vi "setnag_testing.vi"() -> ()   [LabVIEW 2013]
doc: "This example demonstrates temperature control and monitoring.\n\nNote:\nBefore start this VI is it necessary:\n\n- preconfigure some specific parameters that are not supported by this driver (e.g. PV-I/O Type, Linearization type, Alarm Input Values... ) by Quick Codes, or by Eurotherm iTools or by instrument front panel controls\n- enter correct VISA Resource Descriptor, Device Address and Baud Rate into front-panel controls"
uses:
  <vilib>/DAQmx/read.llb/DAQmx Read (Analog DBL 1Chan 1Samp).vi
  <vilib>/Utility/file.llb/Write To Spreadsheet File (string).vi
  <vilib>/DAQmx/miscellaneous.llb/DAQmx Fill In Error Info.vi
panel:
  in  "stop":bool
  in  "Tab Control":enum32{"Setup", "QCM", "SetNag O2 Gauge"}(tab)
  in  "Add comments to the data file here and click anywhere outside the comment box to save. \nThe time at which comment is saved is recorded in the data file.":string
  out "Waveform Chart 2":dbl(graph)
  out "Waveform Chart":cluster{dbl}(graph)
  in  "Baud Rate":i32(ring)=2 items=["2400", "4800", "9600", "19200", "38400", "57600", "115200"]
  in  "Com Port":i32(ring) items=["Com 1", "Com 2", "Com 3", "Com 4", "Com 5", "Com 6", "COM 7", "COM 8", "COM 9", "COM 10", "COM 11", "COM 12", "com 13", "COM 14"]
  out "Torr":dbl
  out "%":dbl
  out "O2 pump voltage (V)":dbl format="%0.2f"
  out "atm":dbl
  # "Configuring Instrument\n \nPlease Wait......\n\nChart will update in 20 sec"
  # "Instructions:\n\nMake sure all instruments are plugged into the correct ports and all instruments are turned on.\n\nRun the Pirani Control software, and make sure the program is configured to save the temp / pressure / gas flow data. \n\nClick the RUN arrow on the toolbar, and wait for instruments to begin recording.\n\nTo end, click \"END PROGRAM AND SAVE DATA\". DO NOT press the STOP button on the toolbar."
  # "COMMENT BOX"
  # "BEFORE YOU RUN THIS VI:\n1. Turn on SetNag and get to 800C\n2. Turn on QCM and plug into corrent COM.\n3. Plug in USB DAQ 6008 and comment to SetNag"
  # "O2 Partial Pressure"
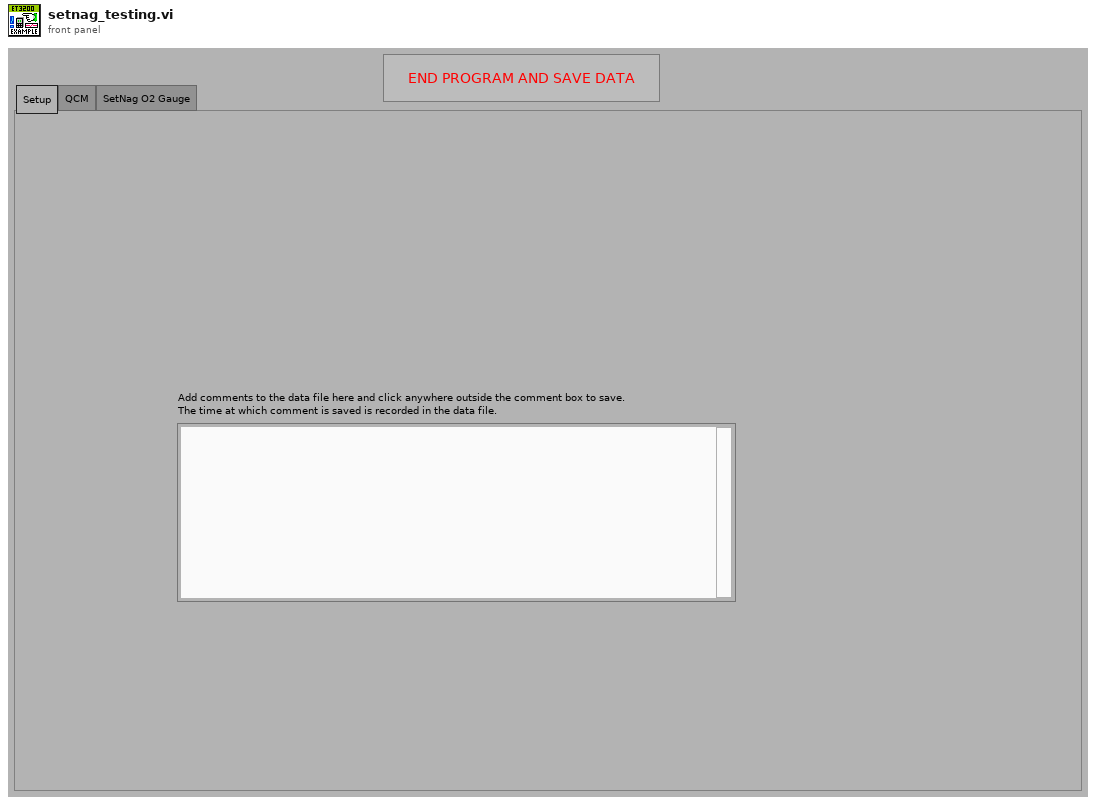
[diagram p1: front panel]
types:
  T1 = enum16{"no parity", "odd parity", "even parity", "mark parity", "space parity"}
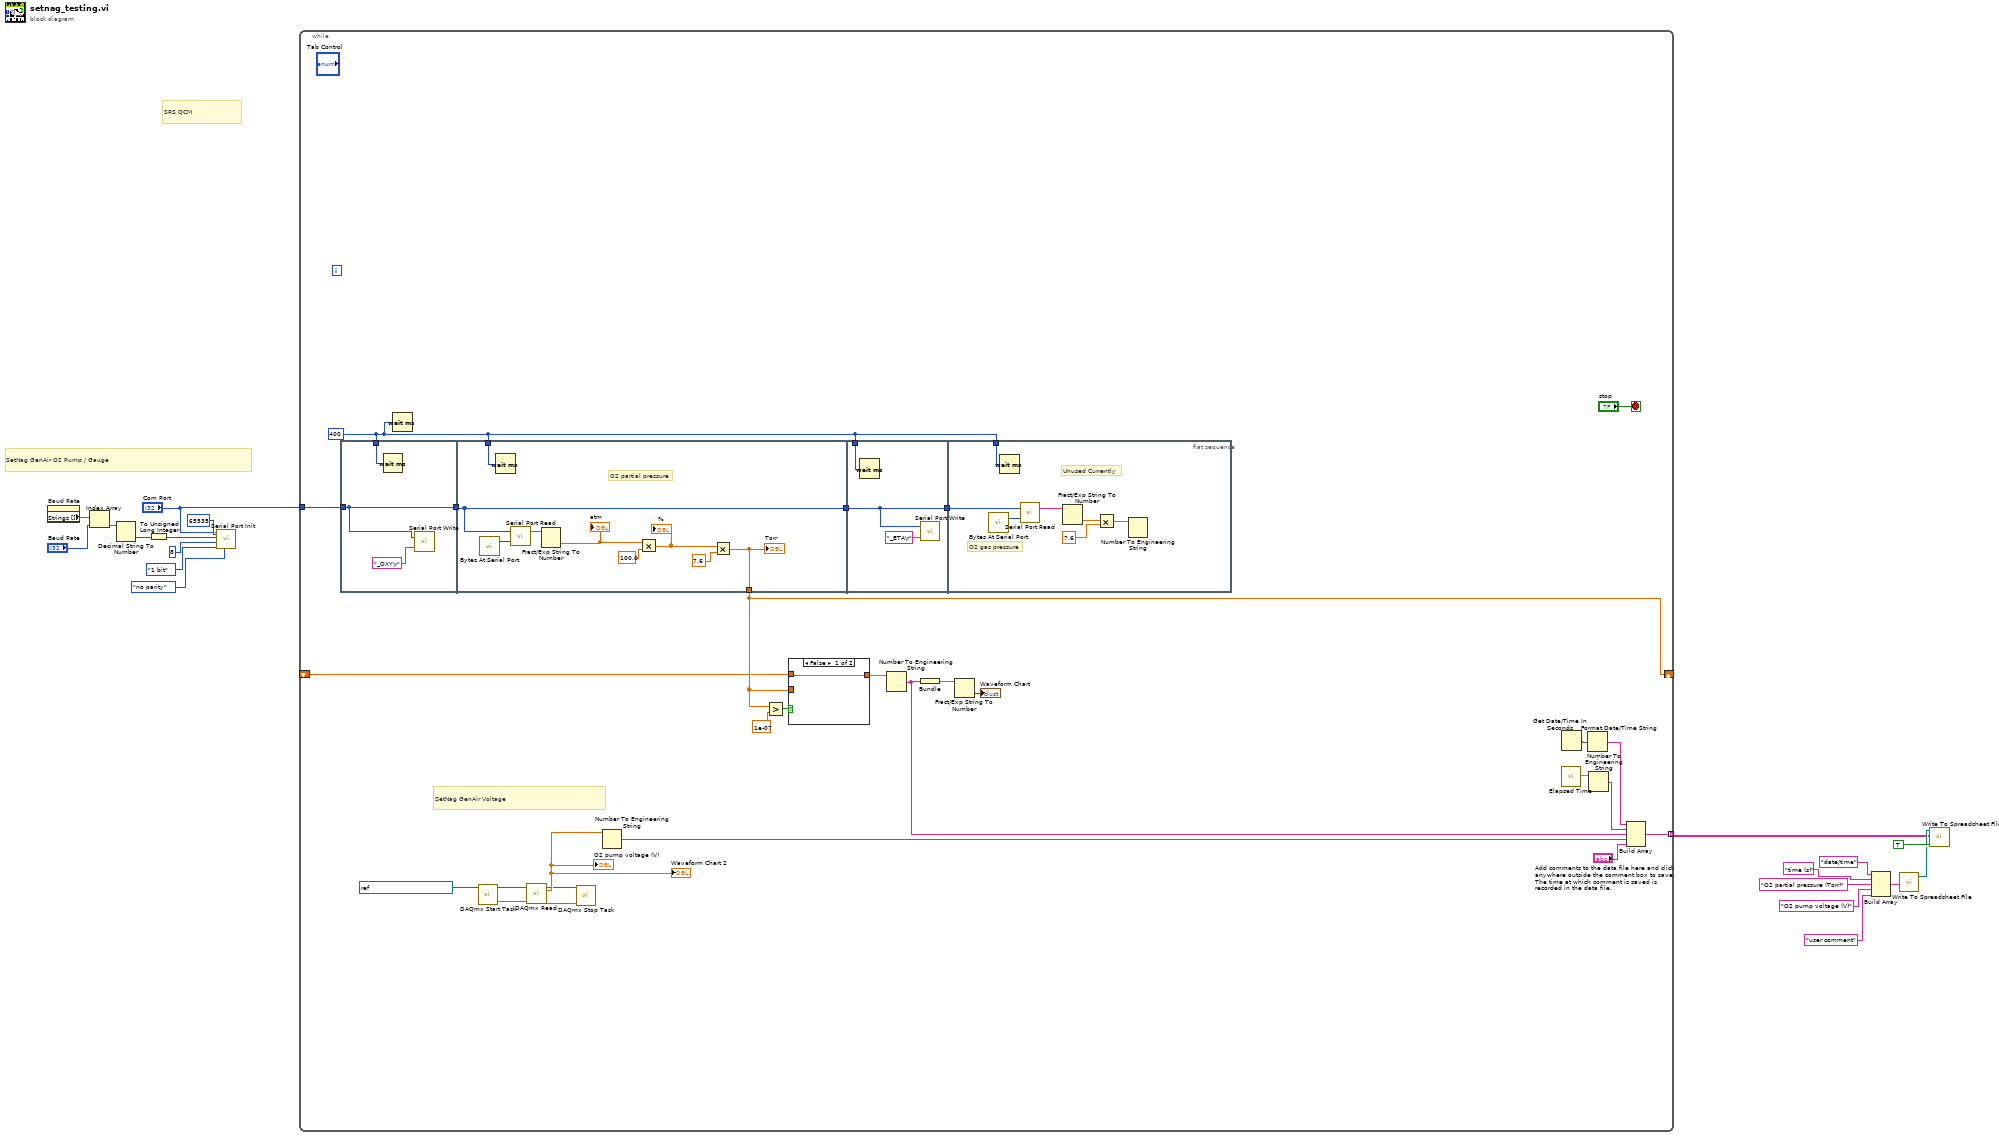
[diagram p0: block diagram]
diagram:
  # "SRS QCM"
  # "SetNag GenAir O2 Pump / Gauge"
  n1 = property on="Baud Rate" class="Ring (strict)"() -> ("Strings []"=w8:string[])  [unwired: 2 in, 2 out]
  n2 = Index Array(array=w8, index="Baud Rate") -> (element=w9:string)
  n3 = Decimal String To Number(string=w9) -> (number=w7:i32)  [unwired: 2 in, 1 out]
  n4 = To Unsigned Long Integer(number=w7) -> (unsigned 32bit integer=w10:u32)
  n5 = call <vilib>:"Serial Port Init.vi"("parity"=T1."no parity", "buffer size"=u16 65535, "stop bits"=enum16{"1 bit", "1.5 bits", "2 bits"}."1 bit", "data bits"=u16 8, "baud rate"=w10, "port number"="Com Port") -> ()  [unwired: 1 in, 1 out]
  n6 = while {
    tunnel: [w45] -> w16 mode=indexing
    tunnel: "Com Port" -> [w39]
    shift-right: [w21] -> _
    shift-left: _ -> [w20]
    stop <- "stop" stop-if-true
    w34 = u32 400 ("milliseconds to wait")
    # "SetNag GenAir Voltage"
    n7 = flat-sequence {
      tunnel: [w49] -> w42
      tunnel: w34 -> [w51]
      tunnel: w39 -> [w49]
      tunnel: w42 -> [w57]
      tunnel: w34 -> [w59]
      tunnel: [w57] -> w36
      tunnel: [w54] -> w21
      tunnel: w36 -> [w62]
      tunnel: [w62] -> w35
      tunnel: w34 -> [w61]
      tunnel: w35 -> [w68]
      tunnel: w34 -> [w67]
      frame #0 {
        n8 = Wait (ms)(milliseconds to wait=w51) -> ()  [unwired: 1 out]
        n9 = call <vilib>:"Serial Port Write.vi"("string to write"="_OXY\r" ("O2 partial press"), "port number"=w49) -> ()  [unwired: 1 out]
      }
      frame #1 {
        # "O2 partial pressure"
        n10 = call <vilib>:"Bytes At Serial Port.vi"() -> ("byte count"=w60:u32)  [unwired: 1 in, 1 out]
        n11 = Wait (ms)(milliseconds to wait=w59) -> ()  [unwired: 1 out]
        n12 = call <vilib>:"Serial Port Read.vi"("requested byte count"=w60, "port number"=w57) -> ("string read"=w58:string)  [unwired: 1 out]
        n13 = Fract/Exp String To Number(string=w58) -> (number=w55:dbl)  [unwired: 3 in, 1 out]
        "atm" <- w55
        n14 = Multiply(x=w55, y=100.0) -> (x*y=w52:dbl)
        "%" <- w52
        n15 = Multiply(x=w52, y=7.6) -> (x*y=w54:dbl)
        "Torr" <- w54
      }
      frame #2 {
        n16 = Wait (ms)(milliseconds to wait=w61) -> ()  [unwired: 1 out]
        n17 = call <vilib>:"Serial Port Write.vi"("string to write"="_ETA\r" ("O2 partial press"), "port number"=w62) -> ()  [unwired: 1 out]
      }
      frame #3 {
        # "Unused Currently"
        # "O2 gas pressure"
        n18 = call <vilib>:"Bytes At Serial Port.vi"() -> ("byte count"=w69:u32)  [unwired: 1 in, 1 out]
        n19 = Wait (ms)(milliseconds to wait=w67) -> ()  [unwired: 1 out]
        n20 = call <vilib>:"Serial Port Read.vi"("requested byte count"=w69, "port number"=w68) -> ("string read"=w70:string)  [unwired: 1 out]
        n21 = Fract/Exp String To Number(string=w70) -> (number=w64:dbl)  [unwired: 3 in, 1 out]
        n22 = Multiply(x=w64, y=7.6) -> (x*y=w65:dbl)
        n23 = Number To Engineering String(4:w65) -> ()  [unwired: 3 in, 1 out]
      }
    }
    n24 = Wait (ms)(milliseconds to wait=w34) -> ()  [unwired: 1 out]
    n25 = call <vilib>:"DAQmx Start Task.vi"("task/channels in"=refnum<k21> "SetNag_Pump_Voltage") -> ("task out"=w32:refnum<k21>, "error out"=w31:errorcluster)  [unwired: 13 in]
    n26 = call-poly <vilib>:"DAQmx Read.vi"("task/channels in"=w32, "error in"=w31) -> ("task out"=w30:refnum<k21>, "data"=w38:dbl, "error out"=w29:errorcluster)  [unwired: 11 in]
    "Waveform Chart 2" <- w38
    "O2 pump voltage (V)" <- w38
    n27 = call <vilib>:"DAQmx Stop Task.vi"("task/channels in"=w30, "error in"=w29) -> ()  [unwired: 12 in, 2 out]
    n28 = Number To Engineering String(4:w38) -> (0:w25:string)  [unwired: 3 in]
    n29 = Greater?(x=w21, y=1e-07) -> (0:w23:bool)
    n30 = case shown="False" w23 {
      tunnel: [w47 w48] -> w22
      tunnel: w21 -> [_ w48]
      tunnel: w20 -> [w47 _]
      frame False {
      }
      frame True {
      }
    }
    n31 = Number To Engineering String(4:w22) -> (0:w28:string)  [unwired: 3 in]
    n32 = Bundle(w28) -> (w37:cluster{string})  [unwired: 1 in]
    n33 = Fract/Exp String To Number(string=w37) -> (number=→"Waveform Chart":cluster{dbl})  [unwired: 3 in, 1 out]
    n34 = call "Elapsed Time"() -> ("Elapsed Time (s)"=w44:dbl)  [unwired: 12 in, 7 out]
    n35 = Get Date/Time In Seconds() -> (seconds since 1Jan1904=w46:timestamp)
    n36 = Format Date/Time String(seconds (now)=w46) -> (date/time string=w26:string)  [unwired: 2 in]
    n37 = Number To Engineering String(4:w44) -> (0:w27:string)  [unwired: 3 in]
    n38 = Build Array(w26, w27, w28, w25, "Add comments to the data file here and click anywhere outside the comment box to save. \nThe time at which comment is saved is recorded in the data file.") -> (w45:string[])
  }
  n39 = Build Array("date/time", "time (s)", "O2 partial pressure (Torr)" ("element"), "O2 pump voltage (V)" ("element"), "user comment" ("element")) -> (w18:string[])
  n40 = call-poly <vilib>:"Write To Spreadsheet File.vi"("1D data"=w18) -> ("new file path (Not A Path if cancelled)"=w17:path)  [unwired: 7 in]
  n41 = call-poly <vilib>:"Write To Spreadsheet File.vi"("append to file? (new file:F)"=TRUE, "2D data"=w16, "file path (dialog if empty)"=w17) -> ()  [unwired: 5 in, 1 out]
